vi "Round To Nearest Multiple.vi"(5 "Round To":dbl=1.0, 11 "Input":dbl) -> (3 "Output":dbl)   [LabVIEW 2012, in "femtoRoboLib.lvlib"]
doc: "Rounds Input to nearest multiple of Round To."
uses:
  femtoRoboLib.lvlib
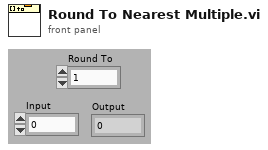
[diagram p1: front panel]
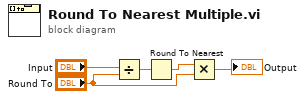
[diagram p0: block diagram]
diagram:
  n1 = Divide(x="Input", y="Round To") -> (x/y=w4:dbl)
  n2 = Round To Nearest(number=w4) -> (nearest integer value=w3:dbl)
  n3 = Multiply(x=w3, y="Round To") -> (x*y=→"Output":dbl)
